vi "RT_main.vi"() -> ()   [LabVIEW 2019]
uses:
  <vilib>/FPGAPlugInAG/myRIO-1900/niLvFpga_Open_myRIO-1900.vi
  <vilib>/rvi/interface/common/dynamic/niFpgaDynamicAddResources.vi
  <vilib>/Utility/error.llb/Error Cluster From Error Code.vi
  <vilib>/rvi/errors/niLvFpgaAdjustHostInterfaceError.vi
  <vilib>/FPGAPlugInAG/Dynamic/niLvFpga_Run_Dynamic.vi
  <vilib>/FPGAPlugInAG/Dynamic/niLvFpga_Abort_Dynamic.vi
  <vilib>/FPGAPlugInAG/Dynamic/niLvFpga_Close_Dynamic.vi
  <vilib>/rvi/interface/nirviOpenFPGA/nirviOpenFPGA.xnode
  FPGA Bitfiles/grzegorzlis_FPGATarget_FPGAmain_Rr4tf5VPCB0.lvbitx
  FPGA_main.vi
  <vilib>/rvi/interface/nirviReadWriteControl/nirviReadWriteControl.xnode
  <vilib>/rvi/interface/nirviMethod/nirviMethod.xnode
  <vilib>/rvi/interface/nirviCloseFPGA/nirviCloseFPGA.xnode
  <vilib>/FPGAPlugInAG/Dynamic/niLvFpga_ReadFifo_Dynamic.vi
  <vilib>/rvi/errors/niLvFpgaMergeErrorWithErrorCode.vi
  NiFpgaLv.dll
  <vilib>/rvi/interface/Simulation/niFpgaSimulationCallBeginRW.vi
panel:
  out "Elements remaining":u32
  out "Waveform Graph":i16[][](graph)
  in  "stop":bool
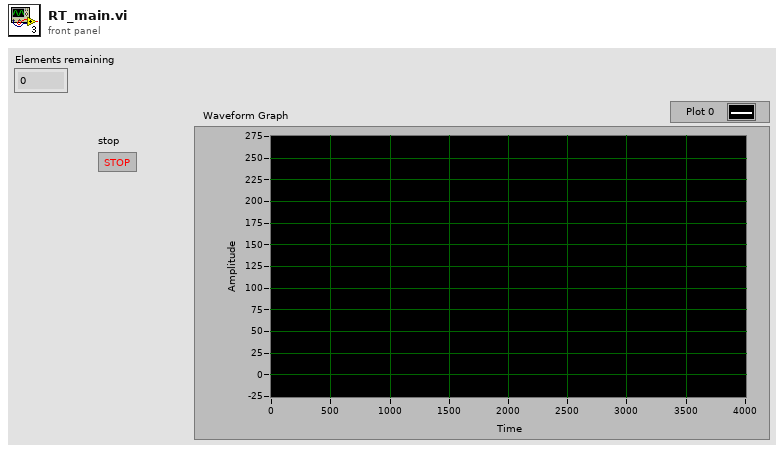
[diagram p1: front panel]
types:
  T1 = cluster{"X_Trigger":i16, "Y_Trigger":i16, "Z_Trigger":i16}
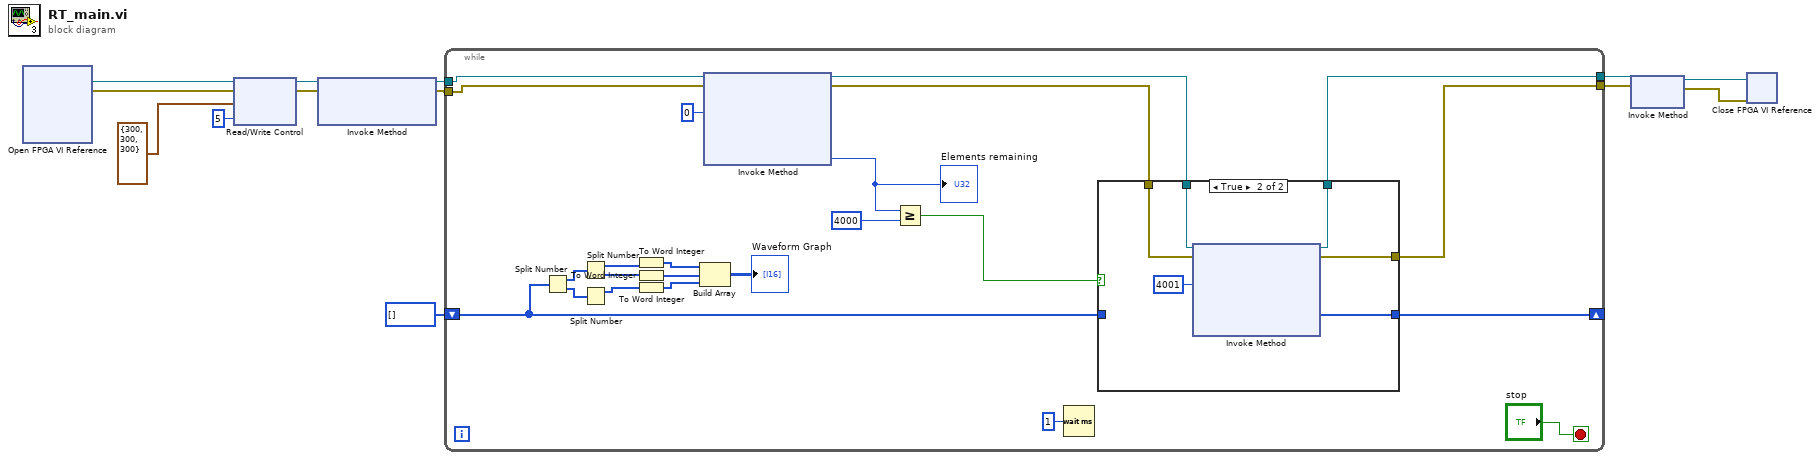
[diagram p0: block diagram]
diagram:
  n1 = xnode "Open FPGA VI Reference"() -> ("FPGA VI Reference Out"=w9:refnum<k20>, "error out"=w8:errorcluster)  [unwired: 2 in]
  n2 = xnode "Read/Write Control"("FPGA VI Reference In"=w9, "error in"=w8, "Trigger"=T1 {"X_Trigger"=300, "Y_Trigger"=300, "Z_Trigger"=300}, "Samples"=i16 5) -> ("FPGA VI Reference Out"=w7:refnum<k20>, "error out"=w6:errorcluster)
  n3 = xnode "Invoke Method"("FPGA VI Reference In"=w7, "error in"=w6) -> ("FPGA VI Reference Out"=w5:refnum<k20>, "error out"=w4:errorcluster)  [unwired: 1 in]
  n4 = while {
    tunnel: [w26] -> w13
    tunnel: [w24] -> w12
    tunnel: w5 -> [w34]
    tunnel: w4 -> [w33]
    shift-right: [w28] -> _
    shift-left: u64[] [] ("Data") -> [w23]
    stop <- "stop" stop-if-true
    n5 = Split Number(x=w23) -> (hi(x)=w21:u32[], lo(x)=w22:u32[])
    n6 = Split Number(x=w21) -> (hi(x)=w16:u16[], lo(x)=w15:u16[])
    n7 = Split Number(x=w22) -> (hi(x)=w14:u16[])  [unwired: 1 out]
    n8 = To Word Integer(number=w16) -> (16bit integer=w19:i16[])
    n9 = To Word Integer(number=w15) -> (16bit integer=w18:i16[])
    n10 = To Word Integer(number=w14) -> (16bit integer=w17:i16[])
    n11 = Build Array(w19, w18, w17) -> (→"Waveform Graph":i16[][])
    n12 = xnode "Invoke Method"("FPGA VI Reference In"=w34, "error in"=w33, "Number of Elements"=u32 0) -> ("FPGA VI Reference Out"=w27:refnum<k20>, "error out"=w25:errorcluster, "Elements Remaining"=w31:u32)  [unwired: 1 in, 1 out]
    "Elements remaining" <- w31
    n13 = Greater Or Equal?(x=w31, y=u32 4000) -> (x >= y?=w29:bool)
    n14 = Wait (ms)(milliseconds to wait=u32 1) -> ()  [unwired: 1 out]
    n15 = case shown="True" w29 {
      tunnel: [w39 w45] -> w28
      tunnel: w23 -> [w39 _]
      tunnel: w27 -> [w38 w43]
      tunnel: [w38 w42] -> w26
      tunnel: w25 -> [w37 w41]
      tunnel: [w37 w40] -> w24
      frame False {
      }
      frame True {
        n16 = xnode "Invoke Method"("FPGA VI Reference In"=w43, "error in"=w41, "Number of Elements"=u32 4001) -> ("FPGA VI Reference Out"=w42:refnum<k20>, "error out"=w40:errorcluster, "Data"=w45:u64[])  [unwired: 1 in, 1 out]
      }
    }
  }
  n17 = xnode "Invoke Method"("FPGA VI Reference In"=w13, "error in"=w12) -> ("FPGA VI Reference Out"=w11:refnum<k20>, "error out"=w10:errorcluster)
  n18 = xnode "Close FPGA VI Reference"("FPGA VI Reference In"=w11, "error in"=w10) -> ()  [unwired: 1 out]
